vi "TIFF Write Encoded Strip.vi"(7 "para3":cluster{}, 8 "error in (no error)":errorcluster, 9 "para2":cluster{}, 10 "para1":cluster{}, 11 "para0":cluster{}) -> (0 "error out":errorcluster, 1 "para2 out":cluster{}, 2 "function return":i32, 3 "para0 out":cluster{})   [LabVIEW 2018]
doc: "LIBTIFF_DLL_IMPEXP tsize_t TIFFWriteEncodedStrip(TIFF*, tstrip_t, tdata_t, tsize_t);\nextern tsize_t TIFFWriteEncodedStrip(TIFF*, tstrip_t, tdata_t, tsize_t);"
uses:
  libtiff3.dll
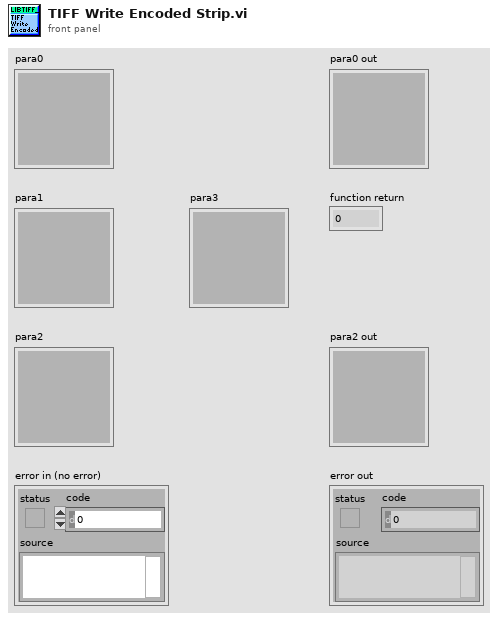
[diagram p1: front panel]
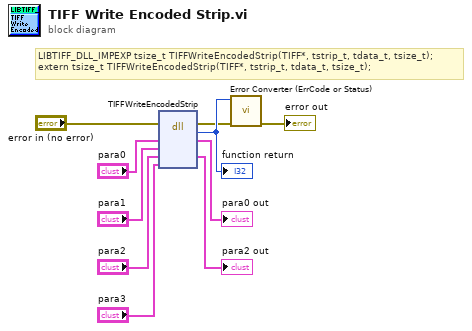
[diagram p0: block diagram]
diagram:
  # "LIBTIFF_DLL_IMPEXP\ttsize_t TIFFWriteEncodedStrip(TIFF*, tstrip_t, tdata_t, tsize_t);\nextern\ttsize_t TIFFWriteEncodedStrip(TIFF*, tstrip_t, tdata_t, tsize_t);"
  n1 = dll-call lib="C:/Users/johan/Downloads/LabVIEW software/LabVIEW software/IX-81 Software/lib/tiff/LibTiffLabview/libtiff3.*" fn="TIFFWriteEncodedStrip"(error in="error in (no error)", "para0"="para0", "para1"="para1", "para2"="para2", "para3"="para3") -> (error out=w2:errorcluster, w10:i32, "para0"=→"para0 out":cluster{}, "para2"=→"para2 out":cluster{})  [unwired: 4 in, 1 out]
  "function return" <- w10
  n2 = call "Error Converter (ErrCode or Status).vi"("error in (no error)"=w2, "error code"=w10) -> ("error out"=→"error out":errorcluster)  [unwired: 9 in]
